vi "Compare_Coordinates_with_Absolute_Presicion-1.vi"(0 "X 1":dbl, 1 "Y 1":dbl, 2 "X 2":dbl, 3 "Y 2":dbl) -> (5 "[OUT] Same coordinates?":bool)   [LabVIEW 2013]
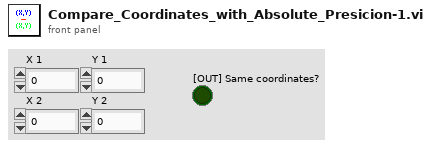
[diagram p1: front panel]
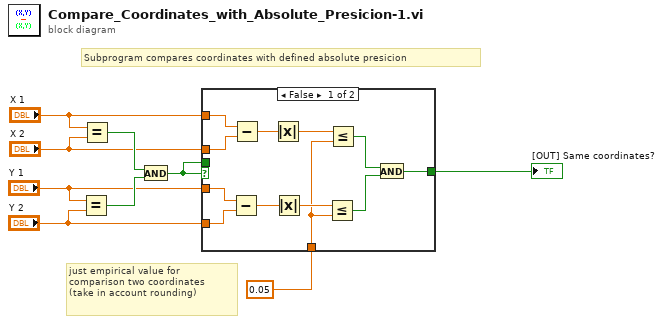
[diagram p0: block diagram]
diagram:
  # "just empirical value for\ncomparison two coordinates\n(take in account rounding)"
  # "Subprogram compares coordinates with defined absolute presicion"
  n1 = Equal?(x="Y 1", y="Y 2") -> (x = y?=w8:bool)
  n2 = Equal?(x="X 1", y="X 2") -> (x = y?=w9:bool)
  n3 = And(x=w9, y=w8) -> (x .and. y?=w7:bool)
  n4 = case shown="False" w7 {
    tunnel: w7 -> [_ w22]
    tunnel: [w10 w22] -> w2
    tunnel: "X 1" -> [w21 _]
    tunnel: "X 2" -> [w20 _]
    tunnel: "Y 1" -> [w19 _]
    tunnel: "Y 2" -> [w18 _]
    tunnel: 0.05 ("Presicion") -> [w13 _]
    frame False {
      n5 = Subtract(x=w19, y=w18) -> (x-y=w16:dbl)
      n6 = Subtract(x=w21, y=w20) -> (x-y=w17:dbl)
      n7 = Absolute Value(x=w17) -> (abs(x)=w14:dbl)
      n8 = Absolute Value(x=w16) -> (abs(x)=w15:dbl)
      n9 = Less Or Equal?(x=w15, y=w13) -> (x <= y?=w11:bool)
      n10 = Less Or Equal?(x=w14, y=w13) -> (x <= y?=w12:bool)
      n11 = And(x=w12, y=w11) -> (x .and. y?=w10:bool)
    }
    frame True {
    }
  }
  "[OUT] Same coordinates?" <- w2
